vi "svfa_Tone Estimation Subroutine G(f) (complex).vi"(4 "N (window length)":i32=512, 5 "window":T1(ring), 6 "frequency":dbl format="%.5e", 7 "three fingers":cluster{"f0":dbl, "df":dbl, "spectrum":cdb[]}={"f0"=0.0, "df"=1.0, "spectrum"=[]} {"spectrum" format="%.2f"; "df" format="%.2f"; "f0" format="%.2f"}) -> (1 "phase [degree]":dbl format="%.2f", 2 "Amplitude":dbl format="%.2f", 3 "G(f)":dbl format="%.2e")   [LabVIEW 2017]
doc: "This is the actual function involved in the Newton-Raphson's root finding loop.\nG(f) is the function to be evaluated. for each iteration, amplitude and phase are also computed."
uses:
  <vilib>/addons/_NISVFA/_Spectrum Processing/subVIs/svfa_Window Frequency Response (double array).vi
  <vilib>/Analysis/baseanly.llb/Complex Dot Product.vi
  <vilib>/addons/_NISVFA/_Spectrum Processing/subVIs/svfa_Rect Window Frequency Response.vi
  <vilib>/addons/_NISVFA/_Spectrum Processing/subVIs/svfa_Cosine Window Coefficients.vi
  <vilib>/Analysis/NI_AALBase.lvlib
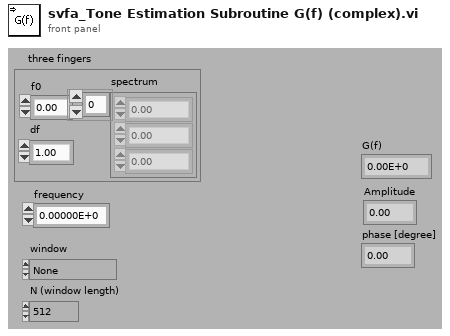
[diagram p1: front panel]
types:
  T1 = enum16{"None ", "Hanning", "Hamming", "Blackman-Harris", "Exact Blackman", "Blackman", "Flat Top", "4 Term B-Harris ", "7 Term B-Harris", "Low Sidelobe"}
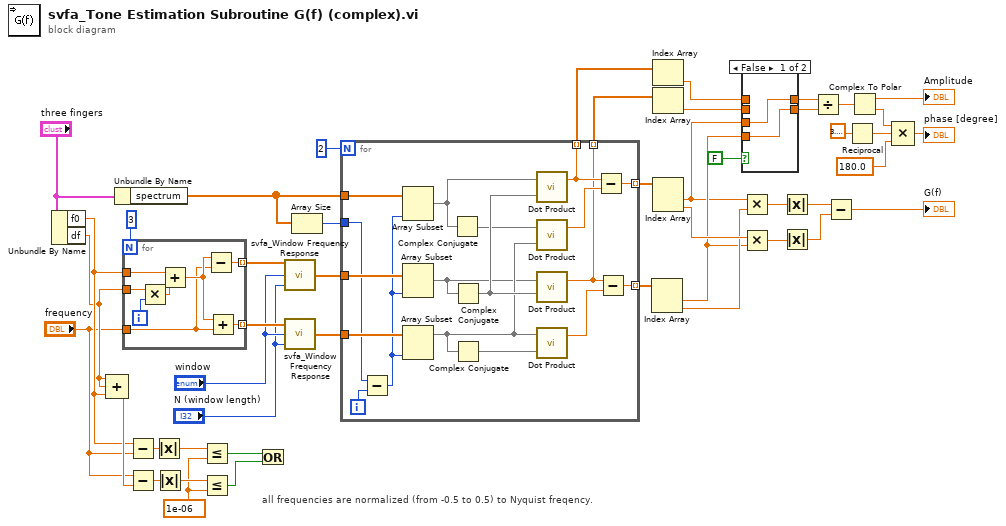
[diagram p0: block diagram]
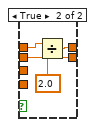
[diagram p2: hidden frame]
diagram:
  w18 = 1e-06 ("y")
  # "all frequencies are normalized (from -0.5 to 0.5) to Nyquist freqency."
  n1 = Unbundle By Name("three fingers") -> ("f0"=w4:dbl, "df"=w3:dbl)
  n2 = Compound Arithmetic op=ADD(w3, w3, w4) -> (w23:dbl)
  n3 = Unbundle By Name("three fingers") -> ("spectrum"=w5:cdb[])
  n4 = for {
    N: 3 -> [_]
    tunnel: w4 -> [w55]
    tunnel: w3 -> [w52]
    tunnel: "frequency" -> [w50]
    tunnel: [w49] -> w38 mode=indexing
    tunnel: [w48] -> w37 mode=indexing
    i -> [w53]
    n5 = Multiply(x=w52, y=w53) -> (x*y=w54:dbl)
    n6 = Add(x=w55, y=w54) -> (x+y=w51:dbl)
    n7 = Subtract(x=w51, y=w50) -> (x-y=w49:dbl)
    n8 = Add(x=w51, y=w50) -> (x+y=w48:dbl)
  }
  n9 = Subtract(x=w4, y="frequency") -> (x-y=w22:dbl)
  n10 = Subtract(x="frequency", y=w23) -> (x-y=w21:dbl)
  n11 = Absolute Value(x=w22) -> (abs(x)=w20:dbl)
  n12 = Absolute Value(x=w21) -> (abs(x)=w19:dbl)
  n13 = Less Or Equal?(x=w20, y=w18) -> (x <= y?=w17:bool)
  n14 = Less Or Equal?(x=w19, y=w18) -> (x <= y?=w7:bool)
  n15 = Or(x=w17, y=w7) -> ()  [unwired: 1 out]
  n16 = call-poly <vilib>:"svfa_Window Frequency Response.vi"("N (window length)"="N (window length)", "window"="window", "f(normalized)"=w38) -> ("H(f)"=w34:cdb[])
  n17 = call-poly <vilib>:"svfa_Window Frequency Response.vi"("N (window length)"="N (window length)", "window"="window", "f(normalized)"=w37) -> ("H(f)"=w35:cdb[])
  n18 = Array Size(array=w5) -> (size(s)=w28:i32)
  n19 = for {
    N: 2 -> [_]
    tunnel: w5 -> [w73]
    tunnel: w35 -> [w71]
    tunnel: w34 -> [w72]
    tunnel: [w68] -> w32 mode=indexing
    tunnel: [w63] -> w31 mode=indexing
    tunnel: w28 -> [w65]
    tunnel: [w58] -> w12 mode=indexing
    tunnel: [w57] -> w11 mode=indexing
    i -> [w56]
    n20 = Subtract(x=w65, y=w56) -> (x-y=w66:i32)
    n21 = Array Subset(array=w73, length=w66) -> (w59:cdb[])  [unwired: 1 in]
    n22 = Array Subset(array=w72, length=w66) -> (w60:cdb[])  [unwired: 1 in]
    n23 = Array Subset(array=w71, length=w66) -> (w61:cdb[])  [unwired: 1 in]
    n24 = Complex Conjugate(1:w59) -> (0:w62:cdb[])
    n25 = Complex Conjugate(1:w60) -> (0:w64:cdb[])
    n26 = Complex Conjugate(1:w61) -> (0:w67:cdb[])
    n27 = call-poly <vilib>:"Dot Product.vi"("Y Vector"=w64, "X Vector"=w59) -> ("X * Y"=w58:cdb)  [unwired: 1 out]
    n28 = call-poly <vilib>:"Dot Product.vi"("Y Vector"=w61, "X Vector"=w62) -> ("X * Y"=w70:cdb)  [unwired: 1 out]
    n29 = call-poly <vilib>:"Dot Product.vi"("Y Vector"=w64, "X Vector"=w60) -> ("X * Y"=w57:cdb)  [unwired: 1 out]
    n30 = call-poly <vilib>:"Dot Product.vi"("Y Vector"=w67, "X Vector"=w61) -> ("X * Y"=w69:cdb)  [unwired: 1 out]
    n31 = Subtract(x=w58, y=w70) -> (x-y=w68:cdb)
    n32 = Subtract(x=w57, y=w69) -> (x-y=w63:cdb)
  }
  n33 = Index Array(array=w31) -> (element #1=w16:cdb, element #2=w25:cdb)  [unwired: 2 in]
  n34 = Index Array(array=w12) -> (element=w9:cdb)  [unwired: 1 in]
  n35 = Index Array(array=w11) -> (element=w10:cdb)  [unwired: 1 in]
  n36 = Index Array(array=w32) -> (element #1=w14:cdb, element #2=w26:cdb)  [unwired: 2 in]
  n37 = case shown="False" FALSE {
    tunnel: w16 -> [w75 _]
    tunnel: [w75 w78] -> w15
    tunnel: w14 -> [w74 _]
    tunnel: [w74 w77] -> w13
    tunnel: w9 -> [_ w79]
    tunnel: w10 -> [_ w78]
    frame False {
    }
    frame True {
      n38 = Divide(x=w79, y=2.0) -> (x/y=w77:cdb)
    }
  }
  n39 = Multiply(x=w14, y=w25) -> (x*y=w30:cdb)
  n40 = Multiply(x=w26, y=w16) -> (x*y=w29:cdb)
  n41 = Absolute Value(x=w30) -> (abs(x)=w46:dbl)
  n42 = Absolute Value(x=w29) -> (abs(x)=w45:dbl)
  n43 = Divide(x=w13, y=w15) -> (x/y=w24:cdb)
  n44 = Subtract(x=w46, y=w45) -> (x-y=→"G(f)":dbl)
  n45 = Reciprocal(x=3.141592653589793) -> (1/x=w42:dbl)
  n46 = Complex To Polar(r * e^(i*theta)=w24) -> (r=→"Amplitude":dbl, theta=w44:dbl)
  n47 = Compound Arithmetic op=MULTIPLY(w44, w42, 180.0 ("Input")) -> (→"phase [degree]":dbl)
